vi "Read Completed Frames Register.vi"(0 "serial channel":fxp<+,3,3>, 5 "serial channel resources":T1) -> (4 "completed frames":u16)   [LabVIEW 2021, in "GettingStarted_Common_148X_FPGA.lvlib"]
uses:
  GettingStarted_Common_148X_FPGA.lvlib
  Types/Serial Channel Resources.ctl
  Types/Single Serial Channel Resources.ctl
  <vilib>/rvi/DataTransferAndStorage/Container/Common/niFpgaContainerExecOnDevCompGetState.vi
  <vilib>/rvi/Emulation/niFpgaEmulationIsFPGAContextNoSignature.vi
  <vilib>/rvi/DataTransferAndStorage/Container/Common/niFpgaContainerGetUniqueNameForEmu.vi
  <vilib>/rvi/Memory/Memory_Emulation/niFpgaMemoryEmulationCacheClearOnFirstRun.vi
  <vilib>/rvi/Memory/Memory_Emulation/nirvimemoryEmulationManagerCache_MakeExclusive.vi
  <vilib>/rvi/Memory/Memory_Emulation/niFpgaMemoryEmulationValidateCache.vi
  <vilib>/rvi/Memory/Memory_Emulation/nirvimemoryEmulationManagerCache_InsertValue.vi
  <vilib>/Utility/error.llb/Clear Errors.vi
  <vilib>/rvi/Memory/Memory_Emulation/nirvimemoryEmulationManagerCache_ReleaseExclusive.vi
  <vilib>/rvi/Memory/Memory_Emulation/nirvimemoryEmulationManagerCache_GetValue.vi
  <vilib>/rvi/Memory/Memory_Emulation/nirvimemoryEmulationManagerCache_SetValue.vi
  <vilib>/rvi/Emulation/niFpgaProcessEmulError.vi
  <vilib>/rvi/Emulation/niFpgaSctlEmulationGetInTimedLoop.vi
  <vilib>/rvi/DataTransferAndStorage/Container/XNode/niFpgaContainer.xnode
  <vilib>/rvi/DataTransferAndStorage/Register/Emulation/niFpgaRegisterEmulationRefIn.vi
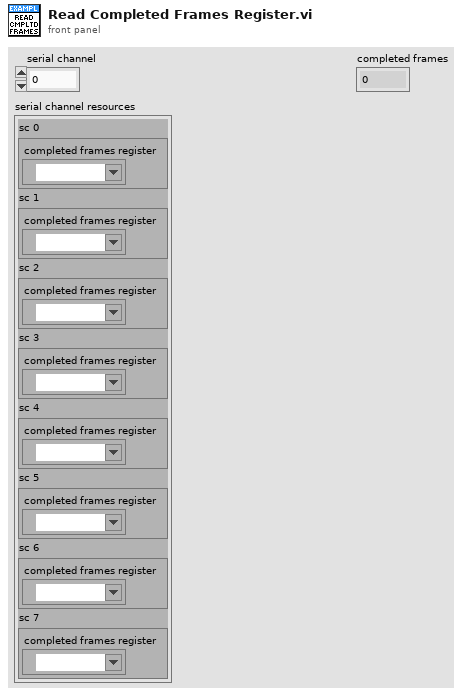
[diagram p1: front panel]
types:
  T1 = typedef "GettingStarted_Common_148X_FPGA.lvlib/Serial Channel Resources.ctl" = cluster{"sc 0":T2, "sc 1":T2, "sc 2":T2, "sc 3":T2, "sc 4":T2, "sc 5":T2, "sc 6":T2, "sc 7":T2}
  T2 = typedef "GettingStarted_Common_148X_FPGA.lvlib/Single Serial Channel Resources.ctl" = cluster{"completed frames register":refnum<k21>}
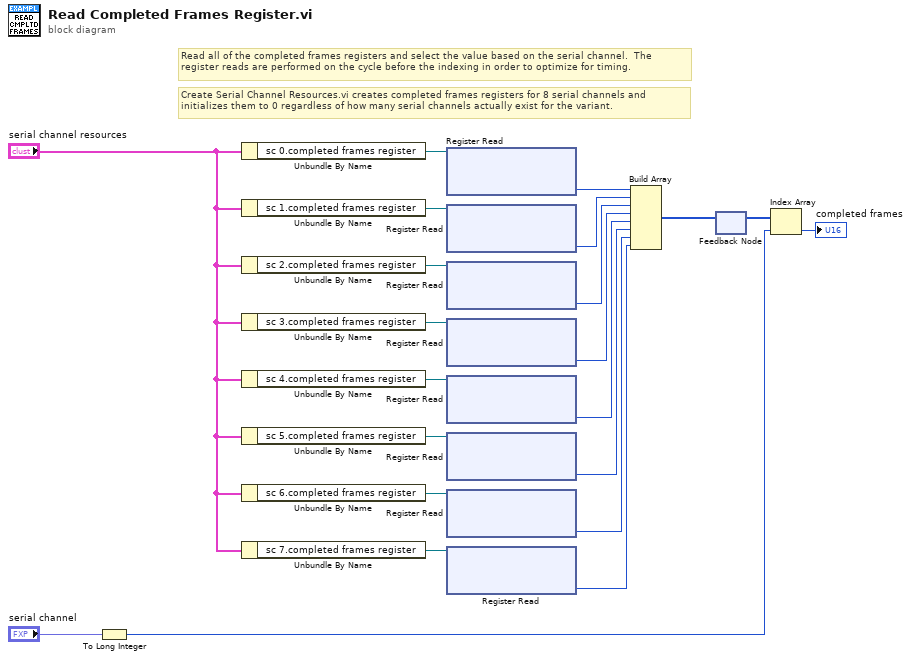
[diagram p0: block diagram]
diagram:
  # "Create Serial Channel Resources.vi creates completed frames registers for 8 serial channels and initializes them to 0 regardless of how many serial channels actually exist for the variant."
  # "Read all of the completed frames registers and select the value based on the serial channel.  The register reads are performed on the cycle before the indexing in order to optimize for timing."
  n1 = To Long Integer(number="serial channel") -> (32bit integer=w21:i32)
  n2 = Unbundle By Name("serial channel resources") -> ("sc 0.completed frames register"=w16:refnum<k21>)
  n3 = Unbundle By Name("serial channel resources") -> ("sc 1.completed frames register"=w15:refnum<k21>)
  n4 = Unbundle By Name("serial channel resources") -> ("sc 2.completed frames register"=w14:refnum<k21>)
  n5 = Unbundle By Name("serial channel resources") -> ("sc 3.completed frames register"=w13:refnum<k21>)
  n6 = Unbundle By Name("serial channel resources") -> ("sc 4.completed frames register"=w12:refnum<k21>)
  n7 = Unbundle By Name("serial channel resources") -> ("sc 5.completed frames register"=w11:refnum<k21>)
  n8 = Unbundle By Name("serial channel resources") -> ("sc 6.completed frames register"=w10:refnum<k21>)
  n9 = Unbundle By Name("serial channel resources") -> ("sc 7.completed frames register"=w9:refnum<k21>)
  n10 = xnode "Register Read"("Register In"=w16) -> ("Data"=w8:u16)  [unwired: 1 out]
  n11 = xnode "Register Read"("Register In"=w15) -> ("Data"=w1:u16)  [unwired: 1 out]
  n12 = xnode "Register Read"("Register In"=w14) -> ("Data"=w2:u16)  [unwired: 1 out]
  n13 = xnode "Register Read"("Register In"=w13) -> ("Data"=w3:u16)  [unwired: 1 out]
  n14 = xnode "Register Read"("Register In"=w12) -> ("Data"=w4:u16)  [unwired: 1 out]
  n15 = xnode "Register Read"("Register In"=w11) -> ("Data"=w5:u16)  [unwired: 1 out]
  n16 = xnode "Register Read"("Register In"=w10) -> ("Data"=w6:u16)  [unwired: 1 out]
  n17 = xnode "Register Read"("Register In"=w9) -> ("Data"=w7:u16)  [unwired: 1 out]
  n18 = Build Array(w8, w1, w2, w3, w4, w5, w6, w7) -> (w22:u16[])
  n19 = feedback #1() -> (w20:u16[])  [unwired: 1 in]
  n20 = feedback-in #1(w22) -> ()
  n21 = Index Array(array=w20, index=w21) -> (element=→"completed frames":u16)
